vi "SysDef.Compile.vi"(8 "error in (no error)":errorcluster, 11 "Device Reference in":T1 format="%.0x") -> (0 "error out":errorcluster, 1 "Refs":T2(array[cluster]) {"VS Refs" format="%.0x"}, 2 "VS References":T3={"Name"="", "CAN"={"Interface"="", "Baud Rate"=0, "Diagnostic Protocol"=enum."GMLAN", "Transport Protocol"=enum."ISO TP - Normal Mode", "Transmit ID"=0, "Receive ID"=2, "Transmit Extension"=1, "Receive Extension"=255, "Receive UUDT ID"=0, "Enable Stream"=TRUE, "VW TP Channel ID"=1, "Fill Frame"=FALSE, "Fill Byte"=0, "Termination"=FALSE, "LIN Cluster"="", "NAD"=8, "IO Mode"=0, "Max DLC"=0, "FD Baud Rate"=2, "Timeout"=1}, "986x"={"Enable"=FALSE, "RIO Device"="", "Bitfile"=path ""}, "Reads"=[], "Frames Lookup"=variant(enum16{"GMLAN", "KWP-2000", "UDS"} enum."GMLAN"), "Writes"=[], "DPIDs"=[], "DPID Lookup"=variant(u32 0), "DTC"={"Descriptor"={"DTC Byte Length"=1, "Status Byte Length"=1, "Add Data Byte Length"=1, "Byte Order"=enum."Motorola"}, "Value.Code"=[], "Value.String"=[], "Value.J2012String"=[], "Status.Code"=[], "Status.String"=[]}, "Created DTCs"=0, "Polls"=[], "Service Channels Status Lookup"=variant, "Trigger Lookup"=variant, "Security"={"Type"=enum."None", "Source DLL Path"=path "", "Target DLL Path"=path "", "Security Level"=1}} {"Writes"."Signals"."Byte Order" items=["Little Endian", "Big Endian"]; "Writes"."Signals"."Data Type" items=["Signed", "Unsigned", "IEEE Float"]; "CAN"."IO Mode" items=["CAN 2.0", "CAN FD", "CAN FD+BRS"]; "CAN"."Fill Byte" format="%.0x"; "CAN"."VW TP Channel ID" format="%.0x"; "CAN"."Receive UUDT ID" format="%.0x"; "CAN"."Receive Extension" format="%.0x"; "CAN"."Transmit Extension" format="%.0x"; "CAN"."Receive ID" format="%.0x"; "CAN"."Transmit ID" format="%.0x"; "Reads"."Signals"."Byte Order" items=["Little Endian", "Big Endian"]; "Reads"."Signals"."Data Type" items=["Signed", "Unsigned", "IEEE Float"]}, 3 "Device Reference out":T1 format="%.0x")   [LabVIEW 2019, in "Diagnostics Addon System Explorer.lvlib"]
uses:
  Diagnostics Addon System Explorer.lvlib
  <vilib>/NI VeriStand/Custom Device API/Custom Device Item Ref.ctl
  Addon Shared/Types/SysDef.Compile.ctl
  Addon Shared/Types/CAN.ctl
  Addon Shared/Types/CAN.Interface.ctl
  Addon Shared/Types/Protocol.ctl
  Addon Shared/Types/Transport.ctl
  Addon Shared/Types/986x.ctl
  Addon Shared/Types/Frame.Compile.ctl
  Addon Shared/Types/Type.ctl
  Addon Shared/Types/Signal.ctl
  Addon Shared/Types/DPID.ctl
  Addon Shared/Types/DPID.Rate.ctl
  Addon Shared/Types/DTC.Settings.ctl
  Addon Shared/Types/DTC.Descriptor.ctl
  Addon Shared/Types/Poll.Compiled.ctl
  Addon Shared/Types/Security.ctl
  Addon Shared/Types/Security.Type.ctl
  Types/FG.Action.ctl
  ID.FG.vi
  Signals.Get.vi
  Type.FG.vi
  ServiceChannels.GetRefs.vi
  SettingChannels.GetRefs.vi
  Addon Shared/SubVIs/Frame.Get.Size.vi
  Addon Shared/SubVIs/LookupID.Create.vi
  DPID.FG.vi
  Security.FG.vi
  Signal.FG.vi
  Frame.GetSignalRefs.vi
  FileDependency.Create.vi
  Addon Shared/SubVIs/Constants.vi
  <vilib>/NI VeriStand/Custom Device Tools/Custom Device Utility Library/NI VeriStand - Search for Item by GUID.vi
  <vilib>/NI VeriStand/Custom Device Tools/Custom Device Utility Library/NI VeriStand - Search for Item by Name.vi
  <vilib>/NI VeriStand/Custom Device API/NI VeriStand - Get Item Children.vi
  <vilib>/NI/NI VeriStand Advanced SysDef API/SysDef API/SysDef.Property.Set.vi
  <vilib>/NI/NI VeriStand Advanced SysDef API/_SubVIs/SysDef.Property.Set.U32.vi
  <vilib>/NI VeriStand/Custom Device API/NI VeriStand - Get Item Property.vi
  <vilib>/NI VeriStand/Custom Device API/Get Item Property (U32).vi
  <vilib>/NI/NI VeriStand Advanced SysDef API/_SubVIs/SysDef.Property.Set.DBL.vi
  <vilib>/NI/NI VeriStand Advanced SysDef API/_SubVIs/SysDef.Property.Set.String.vi
  <vilib>/NI VeriStand/Custom Device API/Get Item Property (Double).vi
  <vilib>/NI VeriStand/Custom Device API/Get Item Property (String).vi
  <vilib>/NI VeriStand/Custom Device API/NI VeriStand - Get Custom Device Channel Data.vi
  <vilib>/NI VeriStand/Custom Device Tools/Custom Device Utility Library/NI VeriStand - Search for All Items by GUID.vi
  Service.EnumToGUID.vi
  FileDependency.Get.Target Path.vi
  <vilib>/Utility/MD5Checksum.llb/MD5Checksum File.vi
  <vilib>/NI/NI VeriStand Advanced SysDef API/_SubVIs/SysDef.Property.Set.DependentFile.vi
  <vilib>/NI/NI VeriStand Advanced SysDef API/SysDef API/SysDef.Property.Remove.vi
  <vilib>/NI/NI VeriStand Advanced SysDef API/_SubVIs/SysDef.Property.Set.U32.Array.vi
  <vilib>/NI VeriStand/Custom Device API/Get Item Property (U32 Array).vi
  Poll.FG.vi
  <vilib>/NI/NI VeriStand Advanced SysDef API/_SubVIs/SysDef.Property.Set.I32.vi
  <vilib>/NI/NI VeriStand Advanced SysDef API/_SubVIs/SysDef.Property.Set.DBL.Array.vi
  <vilib>/NI/NI VeriStand Advanced SysDef API/_SubVIs/SysDef.Property.Set.String.Array.vi
  <vilib>/NI VeriStand/Custom Device API/Get Item Property (I32).vi
  <vilib>/NI VeriStand/Custom Device API/Get Item Property (Double Array).vi
  <vilib>/NI VeriStand/Custom Device API/Get Item Property (String Array).vi
  <vilib>/NI VeriStand/Custom Device API/Get Item Property (Variant).vi
  <vilib>/NI VeriStand/Custom Device API/Get Item Property (Boolean).vi
  <vilib>/NI/NI VeriStand Advanced SysDef API/_SubVIs/SysDef.Property.Set.Variant.vi
  <vilib>/NI/NI VeriStand Advanced SysDef API/_SubVIs/SysDef.Property.Set.Boolean.vi
  <vilib>/NI VeriStand/Custom Device Tools/Custom Device Utility Library/Custom Device Utility Library.lvlib
  Addon Shared/Diagnostics Addon Shared.lvlib
  <vilib>/NI VeriStand/Custom Device API/Custom Device API.lvlib
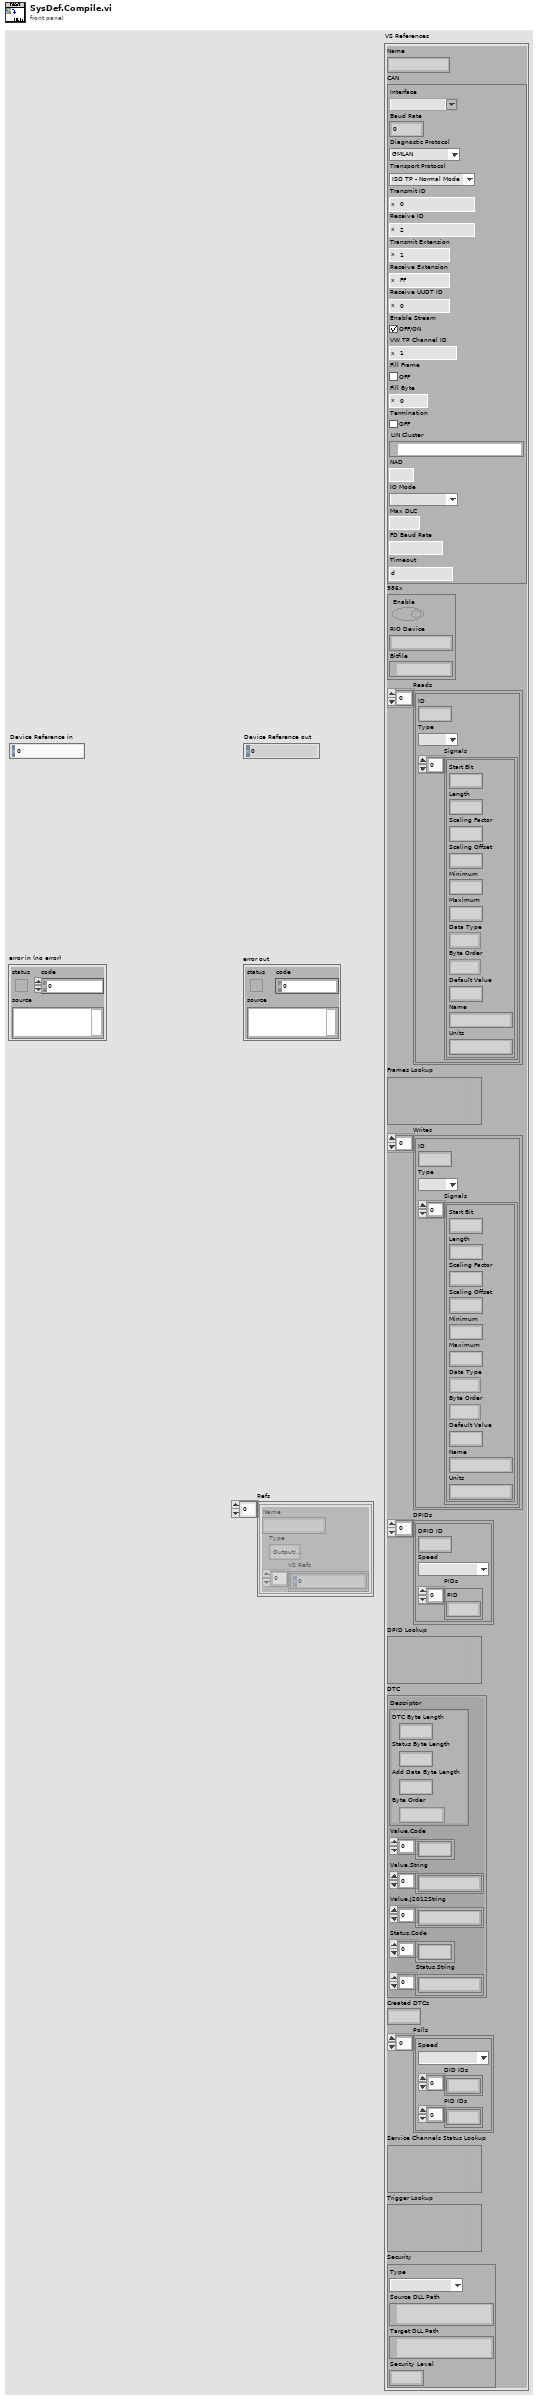
[diagram p1: front panel]
types:
  T1 = typedef "Custom Device API.lvlib/Custom Device Item Ref.ctl" = u64
  T2 = cluster{"Name":string, "Type":enum16{"Output/Write", "Input/Read", "Input/ReadWrite"}, "VS Refs":T1[]}[]
  T3 = typedef "Diagnostics Addon Shared.lvlib/SysDef.Compile.ctl" = cluster{"Name":string, "CAN":T4, "986x":T8, "Reads":T9[], "Frames Lookup":variant, "Writes":T9[], "DPIDs":T12[], "DPID Lookup":variant, "DTC":T14, "Created DTCs":u32, "Polls":T16[], "Service Channels Status Lookup":variant, "Trigger Lookup":variant, "Security":T17}
  T4 = typedef "Diagnostics Addon Shared.lvlib/CAN.ctl" = cluster{"Interface":T5, "Baud Rate":u64, "Diagnostic Protocol":T6, "Transport Protocol":T7, "Transmit ID":u32, "Receive ID":u32, "Transmit Extension":u8, "Receive Extension":u8, "Receive UUDT ID":u32, "Enable Stream":bool, "VW TP Channel ID":u32, "Fill Frame":bool, "Fill Byte":u8, "Termination":bool, "LIN Cluster":refnum<k21>, "NAD":u8, "IO Mode":u32, "Max DLC":u16, "FD Baud Rate":u64, "Timeout":u32}
  T5 = typedef "Diagnostics Addon Shared.lvlib/CAN.Interface.ctl" = string
  T6 = typedef "Diagnostics Addon Shared.lvlib/Protocol.ctl" = enum16{"GMLAN", "KWP-2000", "UDS", "User-Defined"}
  T7 = typedef "Diagnostics Addon Shared.lvlib/Transport.ctl" = enum16{"ISO TP - Normal Mode", "ISO TP - Mixed Mode", "VW TP 2.0", "Diagnostics on IP", "ISO TP LIN"}
  T8 = typedef "Diagnostics Addon Shared.lvlib/986x.ctl" = cluster{"Enable":bool, "RIO Device":string, "Bitfile":path}
  T9 = typedef "Diagnostics Addon Shared.lvlib/Frame.Compile.ctl" = cluster{"ID":u32, "Type":T10, "Signals":T11[]}
  T10 = typedef "Diagnostics Addon Shared.lvlib/Type.ctl" = enum16{"DID", "CDID", "PID", "CPID", "Read Memory", "Write Memory", "IO Control", "Routine Start", "Routine Request", "Routine Stop", "User Defined", "DTC Control", "Clear DTCs", "Read DTCs", "Start DTCs", "DTC Change Count", "Tester Present", "Unlock ECU", "Reset ECU", "Diag Session Control", "Communication Control", "DPID Control", "Poll Control", "Diag CAN Control"}
  T11 = typedef "Diagnostics Addon Shared.lvlib/Signal.ctl" = cluster{"Start Bit":u32, "Length":u32, "Scaling Factor":dbl, "Scaling Offset":dbl, "Minimum":dbl, "Maximum":dbl, "Data Type":u32, "Byte Order":u32, "Default Value":dbl, "Name":string, "Units":string}
  T12 = typedef "Diagnostics Addon Shared.lvlib/DPID.ctl" = cluster{"DPID ID":u8, "Speed":T13, "PIDs":u16[]}
  T13 = typedef "Diagnostics Addon Shared.lvlib/DPID.Rate.ctl" = enum16{"Slow", "Medium", "Fast"}
  T14 = typedef "Diagnostics Addon Shared.lvlib/DTC.Settings.ctl" = cluster{"Descriptor":T15, "Value.Code":dbl[], "Value.String":string[], "Value.J2012String":string[], "Status.Code":dbl[], "Status.String":string[]}
  T15 = typedef "Diagnostics Addon Shared.lvlib/DTC.Descriptor.ctl" = cluster{"DTC Byte Length":i32, "Status Byte Length":i32, "Add Data Byte Length":i32, "Byte Order":enum16{"Motorola", "Intel"}}
  T16 = typedef "Diagnostics Addon Shared.lvlib/Poll.Compiled.ctl" = cluster{"Speed":T13, "DID IDs":u32[], "PID IDs":u32[]}
  T17 = typedef "Diagnostics Addon Shared.lvlib/Security.ctl" = cluster{"Type":T18, "Source DLL Path":path, "Target DLL Path":path, "Security Level":u8}
  T18 = typedef "Diagnostics Addon Shared.lvlib/Security.Type.ctl" = enum16{"None", "SeedKey", "MasterKey"}
  T19 = enum16{"Output/Write", "Input/Read", "Input/ReadWrite"}
  T20 = cluster{"Name":string, "Type":enum16{"Output/Write", "Input/Read", "Input/ReadWrite"}, "VS Refs":T1[]}
  T21 = typedef "Diagnostics Addon System Explorer.lvlib/FG.Action.ctl" = enum16{"Get", "Set"}
  T22 = typedef "Diagnostics Addon System Explorer.lvlib/Service.Export.ctl" = cluster{"Signal.Cmd.Refs":T23[], "Signal.Cmd.Info":T9[], "Signal.Resp.Refs":T23[], "Signal.Resp.Info":T9[], "Trigger.Refs":T23[], "Status.Refs":T23[], "Settings.Refs":T23[]}
  T23 = typedef "Diagnostics Addon System Explorer.lvlib/Frame.Ref.ctl" = cluster{"Type":T10, "ID":u32, "Signal Refs":T1[]}
  T24 = typedef "Custom Device API.lvlib/Custom Device Item Info.ctl" = cluster{"Name":string, "Is Channel":bool, "GUID":string, "Is Waveform":bool}
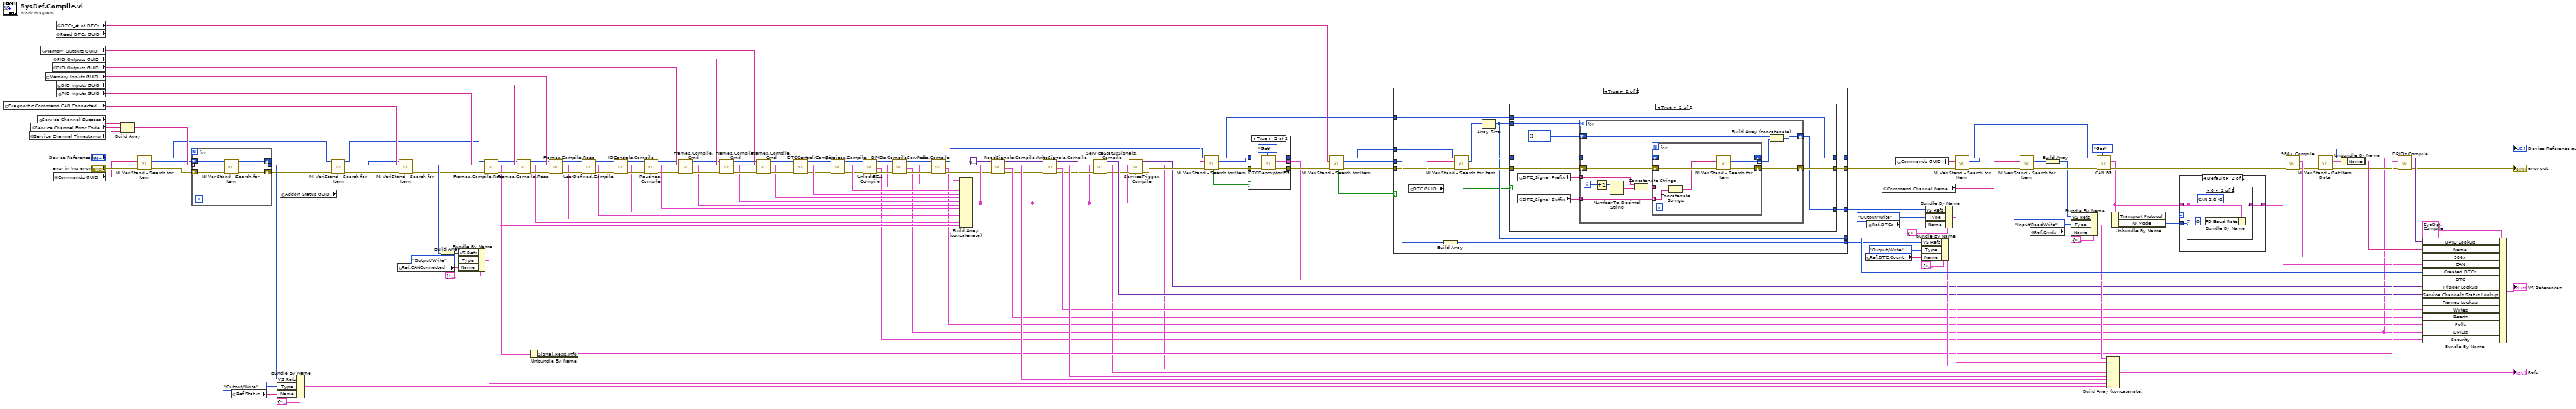
[diagram p0: block diagram]
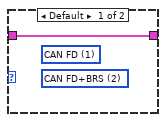
[diagram p3: hidden frame]
diagram:
  n1 = global read "Constants.vi" "Diagnostic Command CAN Connected"() -> (w72:string)
  n2 = global read "Constants.vi" "Service Channel Timestamp"() -> (w14:string)
  n3 = global read "Constants.vi" "Service Channel Error Code"() -> (w15:string)
  n4 = global read "Constants.vi" "Service Channel Success"() -> (w13:string)
  n5 = global read "Constants.vi" "Memory Outputs GUID"() -> (w130:string)
  n6 = global read "Constants.vi" "Memory Inputs GUID"() -> (w129:string)
  n7 = global read "Constants.vi" "DID Outputs GUID"() -> (w110:string)
  n8 = global read "Constants.vi" "PID Outputs GUID"() -> (w149:string)
  n9 = global read "Constants.vi" "Commands GUID"() -> (w63:string)
  n10 = global read "Constants.vi" "Read DTCs GUID"() -> (w153:string)
  n11 = global read "Constants.vi" "DTCs_# of DTCs"() -> (w152:string)
  n12 = global read "Constants.vi" "DID Inputs GUID"() -> (w150:string)
  n13 = global read "Constants.vi" "PID Inputs GUID"() -> (w148:string)
  n14 = Build Array(w13, w15, w14) -> (w114:string[])
  n15 = call-poly <vilib>:"NI VeriStand - Search for Item.vi"("error in"="error in (no error)", "Item GUID"=w63, "Section Ref in"="Device Reference in") -> ("error out"=w6:errorcluster, "Item Ref"=w5:T1, "Section Ref out"=w10:T1)  [unwired: 5 in, 1 out]
  n16 = for {
    tunnel: w114 -> [w157] mode=indexing
    tunnel: [w156] -> w92 mode=indexing
    shift-right: [w155] -> w12
    shift-left: w6 -> [w159]
    shift-right: [w154] -> _
    shift-left: w5 -> [w158]
    n17 = call-poly <vilib>:"NI VeriStand - Search for Item.vi"("error in"=w159, "Item Name"=w157, "Section Ref in"=w158) -> ("error out"=w155:errorcluster, "Item Ref"=w156:T1, "Section Ref out"=w154:T1)  [unwired: 5 in, 1 out]
  }
  n18 = global read "Constants.vi" "Ref.Status"() -> (w100:string)
  n19 = Bundle By Name(cluster=T20 {"Name"="", "Type"=enum."Output/Write", "VS Refs"=[]} ("Group"), "VS Refs"=w92, "Type"=T19."Output/Write", "Name"=w100) -> (w88:T20)
  n20 = global read "Constants.vi" "Addon Status GUID"() -> (w7:string)
  n21 = call-poly <vilib>:"NI VeriStand - Search for Item.vi"("error in"=w12, "Item GUID"=w7, "Section Ref in"=w10) -> ("error out"=w11:errorcluster, "Item Ref"=w8:T1, "Section Ref out"=w9:T1)  [unwired: 5 in, 1 out]
  n22 = global read "Constants.vi" "Ref.CANConnected"() -> (w71:string)
  n23 = call-poly <vilib>:"NI VeriStand - Search for Item.vi"("error in"=w11, "Item Name"=w72, "Section Ref in"=w8) -> ("error out"=w67:errorcluster, "Item Ref"=w69:T1)  [unwired: 5 in, 2 out]
  n24 = Build Array(w69) -> (w68:T1[])
  n25 = Bundle By Name(cluster=T20 {"Name"="", "Type"=enum."Output/Write", "VS Refs"=[]} ("Group"), "VS Refs"=w68, "Type"=T19."Output/Write", "Name"=w71) -> (w62:T20)
  n26 = call "Frames.Compile.Resp.vi"("error in (no error)"=w67, "GUID"=w148, "Section Ref in"=w9) -> ("error out"=w123:errorcluster, "Settings"=w57:T22, "Section Ref out"=w128:T1)  [unwired: 6 in]
  n27 = call "Frames.Compile.Resp.vi"("error in (no error)"=w123, "GUID"=w150, "Section Ref in"=w128) -> ("error out"=w124:errorcluster, "Settings"=w58:T22, "Section Ref out"=w127:T1)  [unwired: 6 in]
  n28 = Unbundle By Name(w57) -> ("Signal.Resp.Info"=w61:T9[])
  n29 = call "Frames.Compile.Resp.vi"("error in (no error)"=w124, "GUID"=w129, "Section Ref in"=w127) -> ("error out"=w108:errorcluster, "Settings"=w59:T22, "Section Ref out"=w109:T1)  [unwired: 6 in]
  n30 = call "UserDefined.Compile.vi"("error in (no error)"=w108, "Section Ref in"=w109) -> ("error out"=w107:errorcluster, "Settings"=w55:T22, "Section Ref out"=w106:T1)  [unwired: 7 in]
  n31 = call "IOControls.Compile.vi"("error in (no error)"=w107, "Section Ref in"=w106) -> ("error out"=w125:errorcluster, "Settings"=w54:T22, "Section Ref out"=w126:T1)  [unwired: 7 in]
  n32 = call "Routines.Compile.vi"("error in (no error)"=w125, "Section Ref in"=w126) -> ("error out"=w48:errorcluster, "Settings"=w53:T22, "Section Ref out"=w47:T1)  [unwired: 7 in]
  n33 = call "Frames.Compile.Cmd.vi"("error in (no error)"=w48, "GUID"=w110, "Section Ref in"=w47) -> ("error out"=w111:errorcluster, "Settings"=w49:T22, "Section Ref out"=w112:T1)  [unwired: 6 in]
  n34 = call "Frames.Compile.Cmd.vi"("error in (no error)"=w111, "GUID"=w149, "Section Ref in"=w112) -> ("error out"=w117:errorcluster, "Settings"=w50:T22, "Section Ref out"=w120:T1)  [unwired: 6 in]
  n35 = call "Frames.Compile.Cmd.vi"("error in (no error)"=w117, "GUID"=w130, "Section Ref in"=w120) -> ("error out"=w118:errorcluster, "Settings"=w51:T22, "Section Ref out"=w119:T1)  [unwired: 6 in]
  n36 = call "DTCControl.Compile.vi"("error in (no error)"=w118, "Section Ref in"=w119) -> ("error out"=w37:errorcluster, "Settings"=w52:T22, "Section Ref out"=w36:T1)  [unwired: 7 in]
  n37 = call "Services.Compile.vi"("error in (no error)"=w37, "Section Ref in"=w36) -> ("error out"=w20:errorcluster, "Settings"=w35:T22[], "Section Ref out"=w21:T1)  [unwired: 7 in]
  n38 = call "UnlockECU.Compile.vi"("error in (no error)"=w20, "Section Ref in"=w21) -> ("error out"=w19:errorcluster, "Security"=w16:T17, "Settings"=w17:T22[], "Section Ref out"=w18:T1)  [unwired: 6 in]
  n39 = call "DPIDs.CompileServices.vi"("error in (no error)"=w19, "Section Ref in"=w18) -> ("error out"=w28:errorcluster, "DPIDs Settings"=w23:T12[], "Settings"=w26:T22, "Section Ref out"=w27:T1)  [unwired: 6 in]
  n40 = call "Polls.Compile.vi"("error in (no error)"=w28, "Section Ref in"=w27) -> ("error out"=w32:errorcluster, "Poll Settings"=w29:T16[], "Service Channels"=w30:T22[], "Section Ref out"=w31:T1)  [unwired: 6 in]
  n41 = Build Array (concatenate)(w30, w26, w17, w35, w52, w51, w50, w49, w53, w54, w55, w59, w58, w57) -> (w40:T22[])
  n42 = call "ReadSignals.Compile.vi"("error in (no error)"=w32, "Settings"=w40, "Lookups in"=variant) -> ("error out"=w46:errorcluster, "Signal Info"=w60:T9[], "Refs"=w89:T20, "Lookups"=w97:variant)  [unwired: 5 in]
  n43 = call "WriteSignals.Compile.vi"("error in (no error)"=w46, "Settings"=w40, "Lookup In"=w97) -> ("error out"=w45:errorcluster, "Signal Info"=w56:T9[], "Refs"=w90:T20, "Lookup"=w96:variant)  [unwired: 5 in]
  n44 = call "ServiceStatusSignals.Compile.vi"("error in (no error)"=w45, "Settings"=w40) -> ("error out"=w42:errorcluster, "Refs"=w44:T20, "Status Lookup"=w43:variant)  [unwired: 7 in]
  n45 = call "ServiceTrigger.Compile.vi"("error in (no error)"=w42, "Settings"=w40) -> ("error out"=w41:errorcluster, "Refs"=w39:T2, "Trigger Lookup"=w38:variant)  [unwired: 7 in]
  n46 = call-poly <vilib>:"NI VeriStand - Search for Item.vi"("error in"=w41, "Item GUID"=w153, "Section Ref in"=w31) -> ("error out"=w144:errorcluster, "Item Ref"=w142:T1, "Section Ref out"=w113:T1, "Found"=w103:bool)  [unwired: 5 in]
  n47 = case shown="True" w103 {
    tunnel: w144 -> [w161 w166]
    tunnel: [w161 w165] -> w143
    tunnel: w142 -> [w160 w164]
    tunnel: [w160 w163] -> w141
    tunnel: [_ w162] -> w140
    frame False {
    }
    frame True {
      n48 = call "DTCDescriptor.FG.vi"("Action"=FG.Action."Get", "error in (no error)"=w166, "Device Item Ref in"=w164) -> ("error out"=w165:errorcluster, "DTC descriptor"=w162:T14, "Device Item Ref out"=w163:T1)  [unwired: 6 in]
    }
  }
  n49 = call-poly <vilib>:"NI VeriStand - Search for Item.vi"("error in"=w143, "Item Name"=w152, "Section Ref in"=w141) -> ("error out"=w146:errorcluster, "Item Ref"=w147:T1, "Section Ref out"=w105:T1, "Found"=w102:bool)  [unwired: 5 in]
  n50 = case shown="True" w102 {
    tunnel: w147 -> [_ w173]
    tunnel: w146 -> [w168 w172]
    tunnel: [_ w183] -> w82
    tunnel: [w168 w182] -> w122
    tunnel: [w169 w181] -> w121
    tunnel: w113 -> [w169 w171]
    tunnel: w105 -> [_ w178]
    tunnel: [_ w175] -> w104
    tunnel: [_ w170] -> w78
    frame False {
    }
    frame True {
      n51 = global read "Constants.vi" "DTC GUID"() -> (w176:string)
      n52 = Build Array(w173) -> (w170:T1[])
      n53 = call-poly <vilib>:"NI VeriStand - Search for Item.vi"("error in"=w172, "Item GUID"=w176, "Section Ref in"=w178) -> ("error out"=w180:errorcluster, "Item Refs"=w179:T1[], "Section Ref out"=w177:T1, "Found"=w174:bool)  [unwired: 5 in]
      n54 = Array Size(array=w179) -> (size(s)=w175:i32)
      n55 = case shown="True" w174 {
        tunnel: [_ w186] -> w183
        tunnel: [w184 w188] -> w182
        tunnel: [w185 w187] -> w181
        tunnel: w171 -> [w185 w187]
        tunnel: w180 -> [w184 w191]
        tunnel: w177 -> [_ w190]
        tunnel: w175 -> [_ w189]
        frame False {
        }
        frame True {
          n56 = global read "Constants.vi" "DTC_Signal Prefix"() -> (w194:string)
          n57 = global read "Constants.vi" "DTC_Signal Suffix"() -> (w193:string[])
          n58 = for {
            N: w189 -> [_]
            tunnel: w190 -> [w206]
            shift-right: [w204] -> w188
            shift-left: w191 -> [w205]
            tunnel: w193 -> [w199]
            tunnel: w194 -> [w198]
            shift-right: [w195] -> w186
            shift-left: T1[] [] -> [w197]
            i -> [w201]
            n59 = Increment(x=w201) -> (x+1=w203:i32)
            n60 = Number To Decimal String(number=w203) -> (decimal integer string=w202:string)  [unwired: 1 in]
            n61 = Concatenate Strings(w198, w202) -> (w200:string)
            n62 = for {
              shift-right: [w213] -> _
              shift-left: w206 -> [w214]
              shift-right: [w211] -> w204
              shift-left: w205 -> [w212]
              tunnel: w199 -> [w210] mode=indexing
              tunnel: w200 -> [w209]
              tunnel: [w207] -> w196 mode=indexing
              n63 = Concatenate Strings(w209, w210) -> (w208:string)
              n64 = call-poly <vilib>:"NI VeriStand - Search for Item.vi"("error in"=w212, "Item Name"=w208, "Section Ref in"=w214) -> ("error out"=w211:errorcluster, "Item Ref"=w207:T1, "Section Ref out"=w213:T1)  [unwired: 5 in, 1 out]
            }
            n65 = Build Array (concatenate)(w197, w196) -> (w195:T1[])
          }
        }
      }
    }
  }
  n66 = global read "Constants.vi" "Ref.DTC.Count"() -> (w80:string)
  n67 = global read "Constants.vi" "Ref.DTCs"() -> (w85:string)
  n68 = global read "Constants.vi" "Command Channel Name"() -> (w74:string)
  n69 = global read "Constants.vi" "Commands GUID"() -> (w151:string)
  n70 = Bundle By Name(cluster=T20 {"Name"="", "Type"=enum."Output/Write", "VS Refs"=[]} ("Group"), "VS Refs"=w78, "Type"=T19."Output/Write", "Name"=w80) -> (w77:T20)
  n71 = Bundle By Name(cluster=T20 {"Name"="", "Type"=enum."Output/Write", "VS Refs"=[]} ("Group"), "VS Refs"=w82, "Type"=T19."Output/Write", "Name"=w85) -> (w83:T20)
  n72 = call-poly <vilib>:"NI VeriStand - Search for Item.vi"("error in"=w122, "Item GUID"=w151, "Section Ref in"=w121) -> ("error out"=w76:errorcluster, "Item Ref"=w75:T1, "Section Ref out"=w33:T1)  [unwired: 5 in, 1 out]
  n73 = call-poly <vilib>:"NI VeriStand - Search for Item.vi"("error in"=w76, "Item Name"=w74, "Section Ref in"=w75) -> ("error out"=w34:errorcluster, "Item Ref"=w73:T1)  [unwired: 5 in, 2 out]
  n74 = global read "Constants.vi" "Ref.Cmds"() -> (w94:string)
  n75 = Build Array(w73) -> (w22:T1[])
  n76 = Bundle By Name(cluster=T20 {"Name"="", "Type"=enum."Output/Write", "VS Refs"=[]} ("Group"), "VS Refs"=w22, "Type"=T19."Input/ReadWrite", "Name"=w94) -> (w91:T20)
  n77 = call "CAN.FG.vi"("Action"=FG.Action."Get", "error in (no error)"=w34, "Device Item Ref in"=w33) -> ("error out"=w139:errorcluster, "Diagnostics Basic Configuration"=w3:T4, "Device Item Ref out"=w138:T1)  [unwired: 6 in]
  n78 = Build Array (concatenate)(w91, w83, w77, w39, w44, w90, w89, w62, w88) -> (→"Refs":T2)
  n79 = Unbundle By Name(w3) -> ("Transport Protocol"=w1:T7, "IO Mode"=w4:u32)
  n80 = case shown="Default" w1 {
    tunnel: w4 -> [_ w218]
    tunnel: w3 -> [w215 w217]
    tunnel: [w215 w216] -> w2
    frame "VW TP 2.0".."ISO TP LIN" {
    }
    frame Default {
      n81 = case shown="0" w218 {
        tunnel: w217 -> [w219 w222]
        tunnel: [w219 w221] -> w216
        frame Default {
          (unwired) u32 2 items=["CAN 2.0", "CAN FD", "CAN FD+BRS"] ("IO Mode")
          (unwired) u32 1 items=["CAN 2.0", "CAN FD", "CAN FD+BRS"] ("IO Mode")
        }
        frame 0 {
          (unwired) u32 0 items=["CAN 2.0", "CAN FD", "CAN FD+BRS"] ("IO Mode")
          n82 = Bundle By Name(cluster=w222, "FD Baud Rate"=u64 0) -> (w221:T4)
        }
      }
    }
  }
  n83 = call "986x.Compile.vi"("error in (no error)"=w139, "Item Ref in"=w138) -> ("error out"=w134:errorcluster, "986x Support"=w137:T8, "Item Ref out"=w133:T1)  [unwired: 7 in]
  n84 = call <vilib>:"NI VeriStand - Get Item Data.vi"("error in (no error)"=w134, "Item Ref in"=w133) -> ("error out"=w25:errorcluster, "Item Info"=w135:T24, "Item Ref out"=→"Device Reference out":T1)  [unwired: 6 in, 1 out]
  n85 = Unbundle By Name(w135) -> ("Name"=w132:string)
  n86 = call "DPIDs.Compile.vi"("error in (no error)"=w25, "PIDs"=w61, "DPIDs"=w23) -> ("error out"=→"error out":errorcluster, "Lookup Table"=w131:variant)  [unwired: 7 in]
  n87 = Bundle By Name(cluster=T3 {"Name"="", "CAN"={"Interface"="", "Baud Rate"=0, "Diagnostic Protocol"=enum."GMLAN", "Transport Protocol"=enum."ISO TP - Normal Mode", "Transmit ID"=0, "Receive ID"=2, "Transmit Extension"=1, "Receive Extension"=255, "Receive UUDT ID"=0, "Enable Stream"=TRUE, "VW TP Channel ID"=1, "Fill Frame"=FALSE, "Fill Byte"=0, "Termination"=FALSE, "LIN Cluster"="", "NAD"=8, "IO Mode"=0, "Max DLC"=0, "FD Baud Rate"=2, "Timeout"=1}, "986x"={"Enable"=FALSE, "RIO Device"="", "Bitfile"=path ""}, "Reads"=[], "Frames Lookup"=variant(enum16{"GMLAN", "KWP-2000", "UDS"} enum."GMLAN"), "Writes"=[], "DPIDs"=[], "DPID Lookup"=variant(u32 0), "DTC"={"Descriptor"={"DTC Byte Length"=1, "Status Byte Length"=1, "Add Data Byte Length"=1, "Byte Order"=enum."Motorola"}, "Value.Code"=[], "Value.String"=[], "Value.J2012String"=[], "Status.Code"=[], "Status.String"=[]}, "Created DTCs"=0, "Polls"=[], "Service Channels Status Lookup"=variant, "Trigger Lookup"=variant, "Security"={"Type"=enum."None", "Source DLL Path"=path "", "Target DLL Path"=path "", "Security Level"=1}} ("VS References"), "DPID Lookup"=w131, "Name"=w132, "986x"=w137, "CAN"=w2, "Created DTCs"=w104, "DTC"=w140, "Trigger Lookup"=w38, "Service Channels Status Lookup"=w43, "Frames Lookup"=w96, "Writes"=w56, "Reads"=w60, "Polls"=w29, "DPIDs"=w23, "Security"=w16) -> (→"VS References":T3)
